vi "sftp_unlink.vi"() -> ()   [LabVIEW 2013]
doc: "Illustrates how to remove a file on a SSH server."
uses:
  libssh2/libssh2_init_default.vi
  libssh2/libssh2_session_handshake_tcp.vi
  libssh2/libssh2.lvlib
panel:
  in  "file":string="/"
  out "error out":errorcluster
  in  "password":string
  in  "username":string
  in  "hostname":string
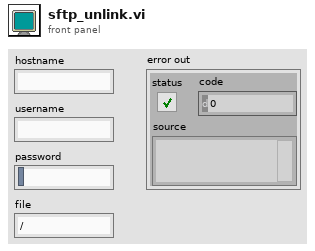
[diagram p1: front panel]
types:
  T1 = typedef "libssh2.lvlib/Session Refnum.ctl" = refnum<k1>
  T2 = typedef "libssh2.lvlib/SFTP Refnum.ctl" = refnum<k1>
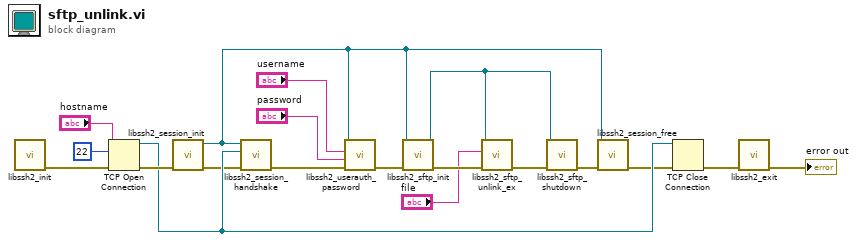
[diagram p0: block diagram]
diagram:
  n1 = call-poly "libssh2_init.vi"() -> ("error out"=w18:errorcluster)  [unwired: 11 in]
  n2 = TCP Open Connection(address="hostname", remote port or service name=u16 22, error in (no error)=w18) -> (connection ID=w16:refnum<k5>, error out=w17:errorcluster)  [unwired: 2 in]
  n3 = call "libssh2_session_init.vi"("error in (no error)"=w17) -> ("error out"=w15:errorcluster, "session"=w8:T1)  [unwired: 9 in]
  n4 = call-poly "libssh2_session_handshake.vi"("error in (no error)"=w15, "tcp connection"=w16, "session"=w8) -> ("error out"=w19:errorcluster)  [unwired: 8 in]
  n5 = call "libssh2_userauth_password.vi"("error in (no error)"=w19, "password"="password", "username"="username", "session"=w8) -> ("error out"=w12:errorcluster)  [unwired: 7 in]
  n6 = call "libssh2_sftp_init.vi"("error in (no error)"=w12, "session"=w8) -> ("error out"=w4:errorcluster, "sftp"=w3:T2)  [unwired: 8 in]
  n7 = call "libssh2_sftp_unlink_ex.vi"("error in (no error)"=w4, "file"="file", "sftp"=w3) -> ("error out"=w1:errorcluster)  [unwired: 8 in]
  n8 = call "libssh2_sftp_shutdown.vi"("error in (no error)"=w1, "sftp"=w3) -> ("error out"=w5:errorcluster)  [unwired: 9 in]
  n9 = call "libssh2_session_free.vi"("error in (no error)"=w5, "session"=w8) -> ("error out"=w7:errorcluster)  [unwired: 9 in]
  n10 = TCP Close Connection(connection ID=w16, error in (no error)=w7) -> (error out=w6:errorcluster)  [unwired: 1 in, 1 out]
  n11 = call "libssh2_exit.vi"("error in (no error)"=w6) -> ("error out"=→"error out":errorcluster)  [unwired: 10 in]
